vi "Set Channel Configurations.vi"(8 "error in (no error)":errorcluster, 9 "Tx Channel Configuration":refnum<class "Configuration.lvclass">, 10 "Rx Channel Configuration":refnum<class "Configuration.lvclass">, 11 "Component Configuration in":refnum<class "Component Configurations.lvclass">) -> (0 "error out":errorcluster, 3 "Component Configuration out":refnum<class "Component Configurations.lvclass">)   [LabVIEW 2017, in "DSF Core.lvlib" / "Component Configurations.lvclass"]
uses:
  Component Configurations.lvclass
  Configuration/Configuration.lvclass
  Component Configurations.lvclass/Component Configurations.ctl
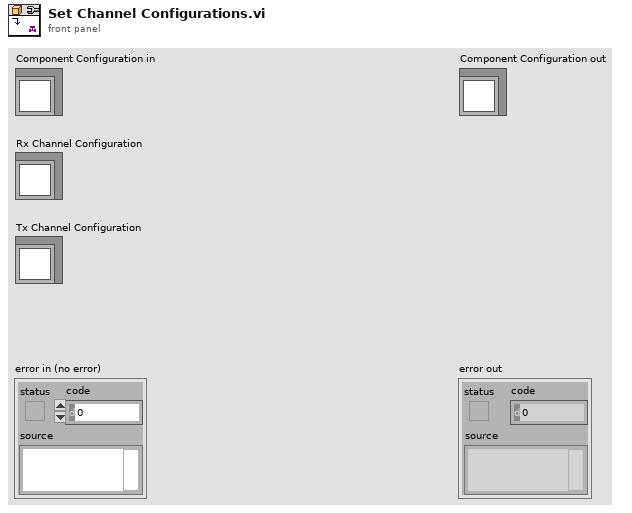
[diagram p1: front panel]
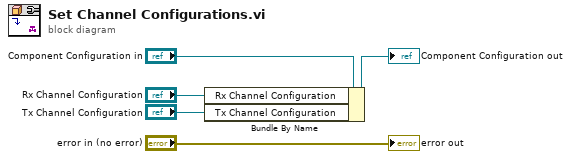
[diagram p0: block diagram]
diagram:
  n1 = Bundle By Name(cluster="Component Configuration in", "Rx Channel Configuration"="Rx Channel Configuration", "Tx Channel Configuration"="Tx Channel Configuration") -> (→"Component Configuration out":refnum<class "Component Configurations.lvclass">)
  "error out" <- "error in (no error)"
